vi "QCP_Set_DBL.vi"(0 "QCP Data Block In":T1, 1 "QCP Name":string, 2 "Value In":dbl) -> (7 "QCP Data Block Out":T1)   [LabVIEW 2015]
uses:
  <userlib>/836 Library/System/QCP Support Code/QCP Data Block.ctl
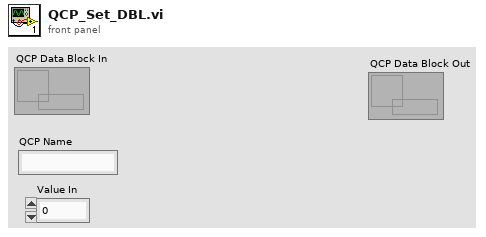
[diagram p1: front panel]
types:
  T1 = typedef "QCP Data Block.ctl" = refnum<data-value>
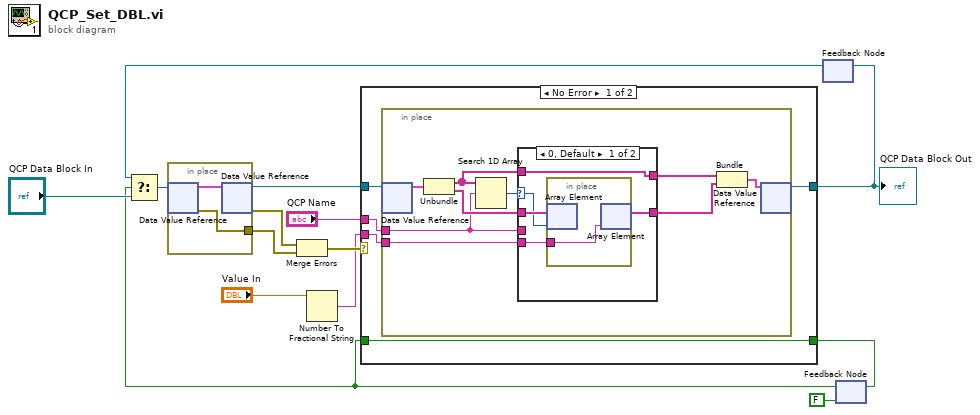
[diagram p0: block diagram]
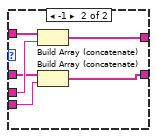
[diagram p2: hidden frame]
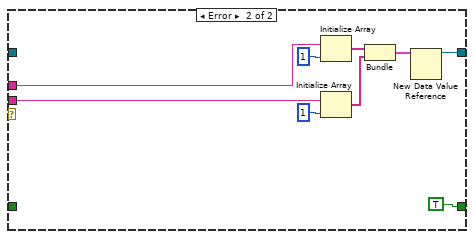
[diagram p3: hidden frame]
diagram:
  n1 = Number To Fractional String(number="Value In") -> (F-format string=w2:string)  [unwired: 3 in]
  n2 = feedback #1() -> (w3:T1)  [unwired: 1 in]
  n3 = feedback #2(FALSE) -> (w4:bool)
  n4 = Select(t=w3, s=w4, f="QCP Data Block In") -> (s? t:f=w5:T1)
  n5 = in-place {
    in-place-border: [w15] -> w13
    n6 = in-place-dvr #3(w5) -> (w16:cluster{string[], string[]}, w15:errorcluster)
    n7 = in-place-dvr #3(w16) -> (w11:T1, w14:errorcluster)
  }
  n8 = Merge Errors(w14, w13) -> (w12:errorcluster)
  n9 = case shown="No Error" w12 {
    tunnel: [w21 w45] -> w9
    tunnel: w11 -> [w20 _]
    tunnel: "QCP Name" -> [w19 w51]
    tunnel: [w18 TRUE] -> w8
    tunnel: w4 -> [w18 _]
    tunnel: w2 -> [w17 w43]
    frame No Error {
      n10 = in-place {
        in-place-border: w19 -> [w23]
        in-place-border: w17 -> [w22]
        n11 = in-place-dvr #4(w20) -> (w30:cluster{string[], string[]})  [unwired: 1 out]
        n12 = Unbundle(w30) -> (w26:string[], w27:string[])
        n13 = Search 1D Array(1D array=w26, element=w23) -> (index of element=w28:i32)  [unwired: 1 out]
        n14 = case shown="0, Default" w28 {
          selector: w28 -> [w33 _]
          tunnel: w23 -> [_ w42]
          tunnel: [w35 w41] -> w25
          tunnel: w22 -> [w32 w40]
          tunnel: [w31 w39] -> w24
          tunnel: w27 -> [w34 w38]
          tunnel: w26 -> [w35 w37]
          frame 0, Default {
            n15 = in-place {
              in-place-border: w32 -> [w36]
              n16 = in-place-array #5(w34, w33) -> ()  [unwired: 1 out]
              n17 = in-place-array #5(w36) -> (w31:string[])  [unwired: 1 out]
            }
          }
          frame -1 {
            n18 = Build Array (concatenate)(w37, w42) -> (w41:string[])
            n19 = Build Array (concatenate)(w38, w40) -> (w39:string[])
          }
        }
        n20 = Bundle(w25, w24) -> (w29:cluster{string[], string[]})  [unwired: 1 in]
        n21 = in-place-dvr #4(w29) -> (w21:T1)  [unwired: 1 out]
      }
    }
    frame Error {
      n22 = Initialize Array(w51, 1 ("dimension size")) -> (w47:string[])
      n23 = Initialize Array(w43, 1 ("dimension size")) -> (w48:string[])
      n24 = Bundle(w47, w48) -> (w46:cluster{string[], string[]})  [unwired: 1 in]
      n25 = New Data Value Reference(data value=w46) -> (data value reference=w45:refnum<data-value>)  [unwired: 1 in, 1 out]
    }
  }
  "QCP Data Block Out" <- w9
  n26 = feedback-in #1(w9) -> ()
  n27 = feedback-in #2(w8) -> ()
